vi "Load Symbols.vi"() -> (3 "Symbols":T1[](array[typedef]))   [LabVIEW 2017, in "Test Executive View.lvclass"]
uses:
  <vilib>/gpm_packages/@cs/Test-executive-builder/Example/Application/Test Executive View/Test Executive View/Test Executive View.lvclass
  <vilib>/gpm_packages/@cs/Test-executive-builder/Source/Application Dependencies/Tree Symbol.ctl
  <vilib>/picture/picture.llb/imagedata.ctl
panel:
  out "Array":bool[](array[boolean])
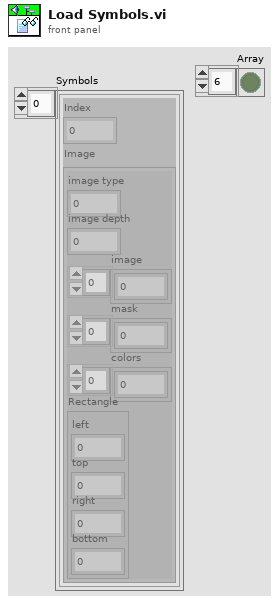
[diagram p1: front panel]
types:
  T1 = typedef "Tree Symbol.ctl" = cluster{"Index":i32, "Image":T2}
  T2 = typedef "imagedata.ctl" = cluster{"image type":i32, "image depth":i32, "image":u8[], "mask":u8[], "colors":u32[], "Rectangle":cluster{"left":i16, "top":i16, "right":i16, "bottom":i16}}
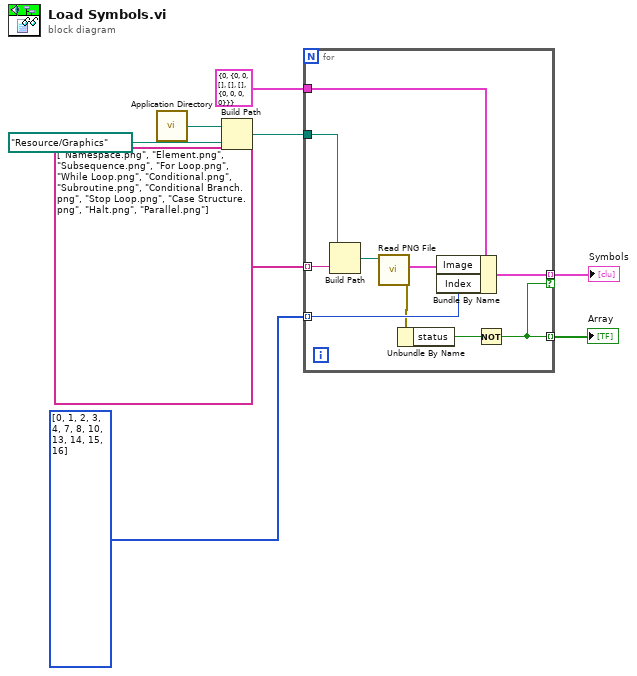
[diagram p0: block diagram]
diagram:
  n1 = call <vilib>:"Application Directory.vi"() -> ("Application Directory"=w8:path)
  n2 = Build Path(base path=w8, name or relative path=path "Resource/Graphics") -> (appended path=w4:path)
  n3 = for {
    tunnel: string[] ["Namespace.png", "Element.png", "Subsequence.png", "For Loop.png", "While Loop.png", "Conditional.png", "Subroutine.png", "Conditional Branch.png", "Stop Loop.png", "Case Structure.png", "Halt.png", "Parallel.png"] -> [w17] mode=indexing
    tunnel: i32[] [0, 1, 2, 3, 4, 7, 8, 10, 13, 14, 15, 16] -> [w13] mode=indexing
    tunnel: w4 -> [w18]
    tunnel: T1 {"Index"=0, "Image"={"image type"=0, "image depth"=0, "image"=[], "mask"=[], "colors"=[], "Rectangle"={"left"=0, "top"=0, "right"=0, "bottom"=0}}} ("Symbol") -> [w15]
    tunnel: [w12] -> w2 mode=indexing if=w9
    tunnel: [w9] -> w1 mode=indexing
    n4 = Build Path(base path=w18, name or relative path=w17) -> (appended path=w16:path)
    n5 = call <vilib>:"Read PNG File.vi"("path to PNG file"=w16) -> ("error out"=w11:errorcluster, "image data"=w14:T2)  [unwired: 8 in, 1 out]
    n6 = Unbundle By Name(w11) -> ("status"=w10:bool)
    n7 = Bundle By Name(cluster=w15, "Image"=w14, "Index"=w13) -> (w12:T1)
    n8 = Not(x=w10) -> (.not. x?=w9:bool)
  }
  "Symbols" <- w2
  "Array" <- w1
